vi "wait_init_04.vi"   [LabVIEW 2011]
uses:
  wait_globals.vi
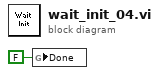
[diagram p0: block diagram]
diagram:
  n1 = global write "wait_globals.vi" "Done"(FALSE ("Done")) -> ()
